vi "Format Container Into String Docs.vi"() -> ()   [LabVIEW 2015]
panel:
  out "resulting string":string
  out "resulting string":string
  out "error out":errorcluster
  out "resulting string":string
  out "resulting string":string
  out "resulting string":string
  out "resulting string":string
  out "resulting string":string
  out "resulting string":string
  out "resulting string":string
  out "resulting string":string
  out "resulting string":string
  out "resulting string":string
  out "resulting string":string
  out "resulting string":string
  out "resulting string":string
  out "resulting string":string
  out "resulting string":string
  out "resulting string":string
  out "resulting string":string
  out "resulting string":string
  out "resulting string":string
  out "resulting string":string
  out "resulting string":string
  out "resulting string":string
  out "resulting string":string
  out "resulting string":string
  out "resulting string":string
  out "resulting string":string
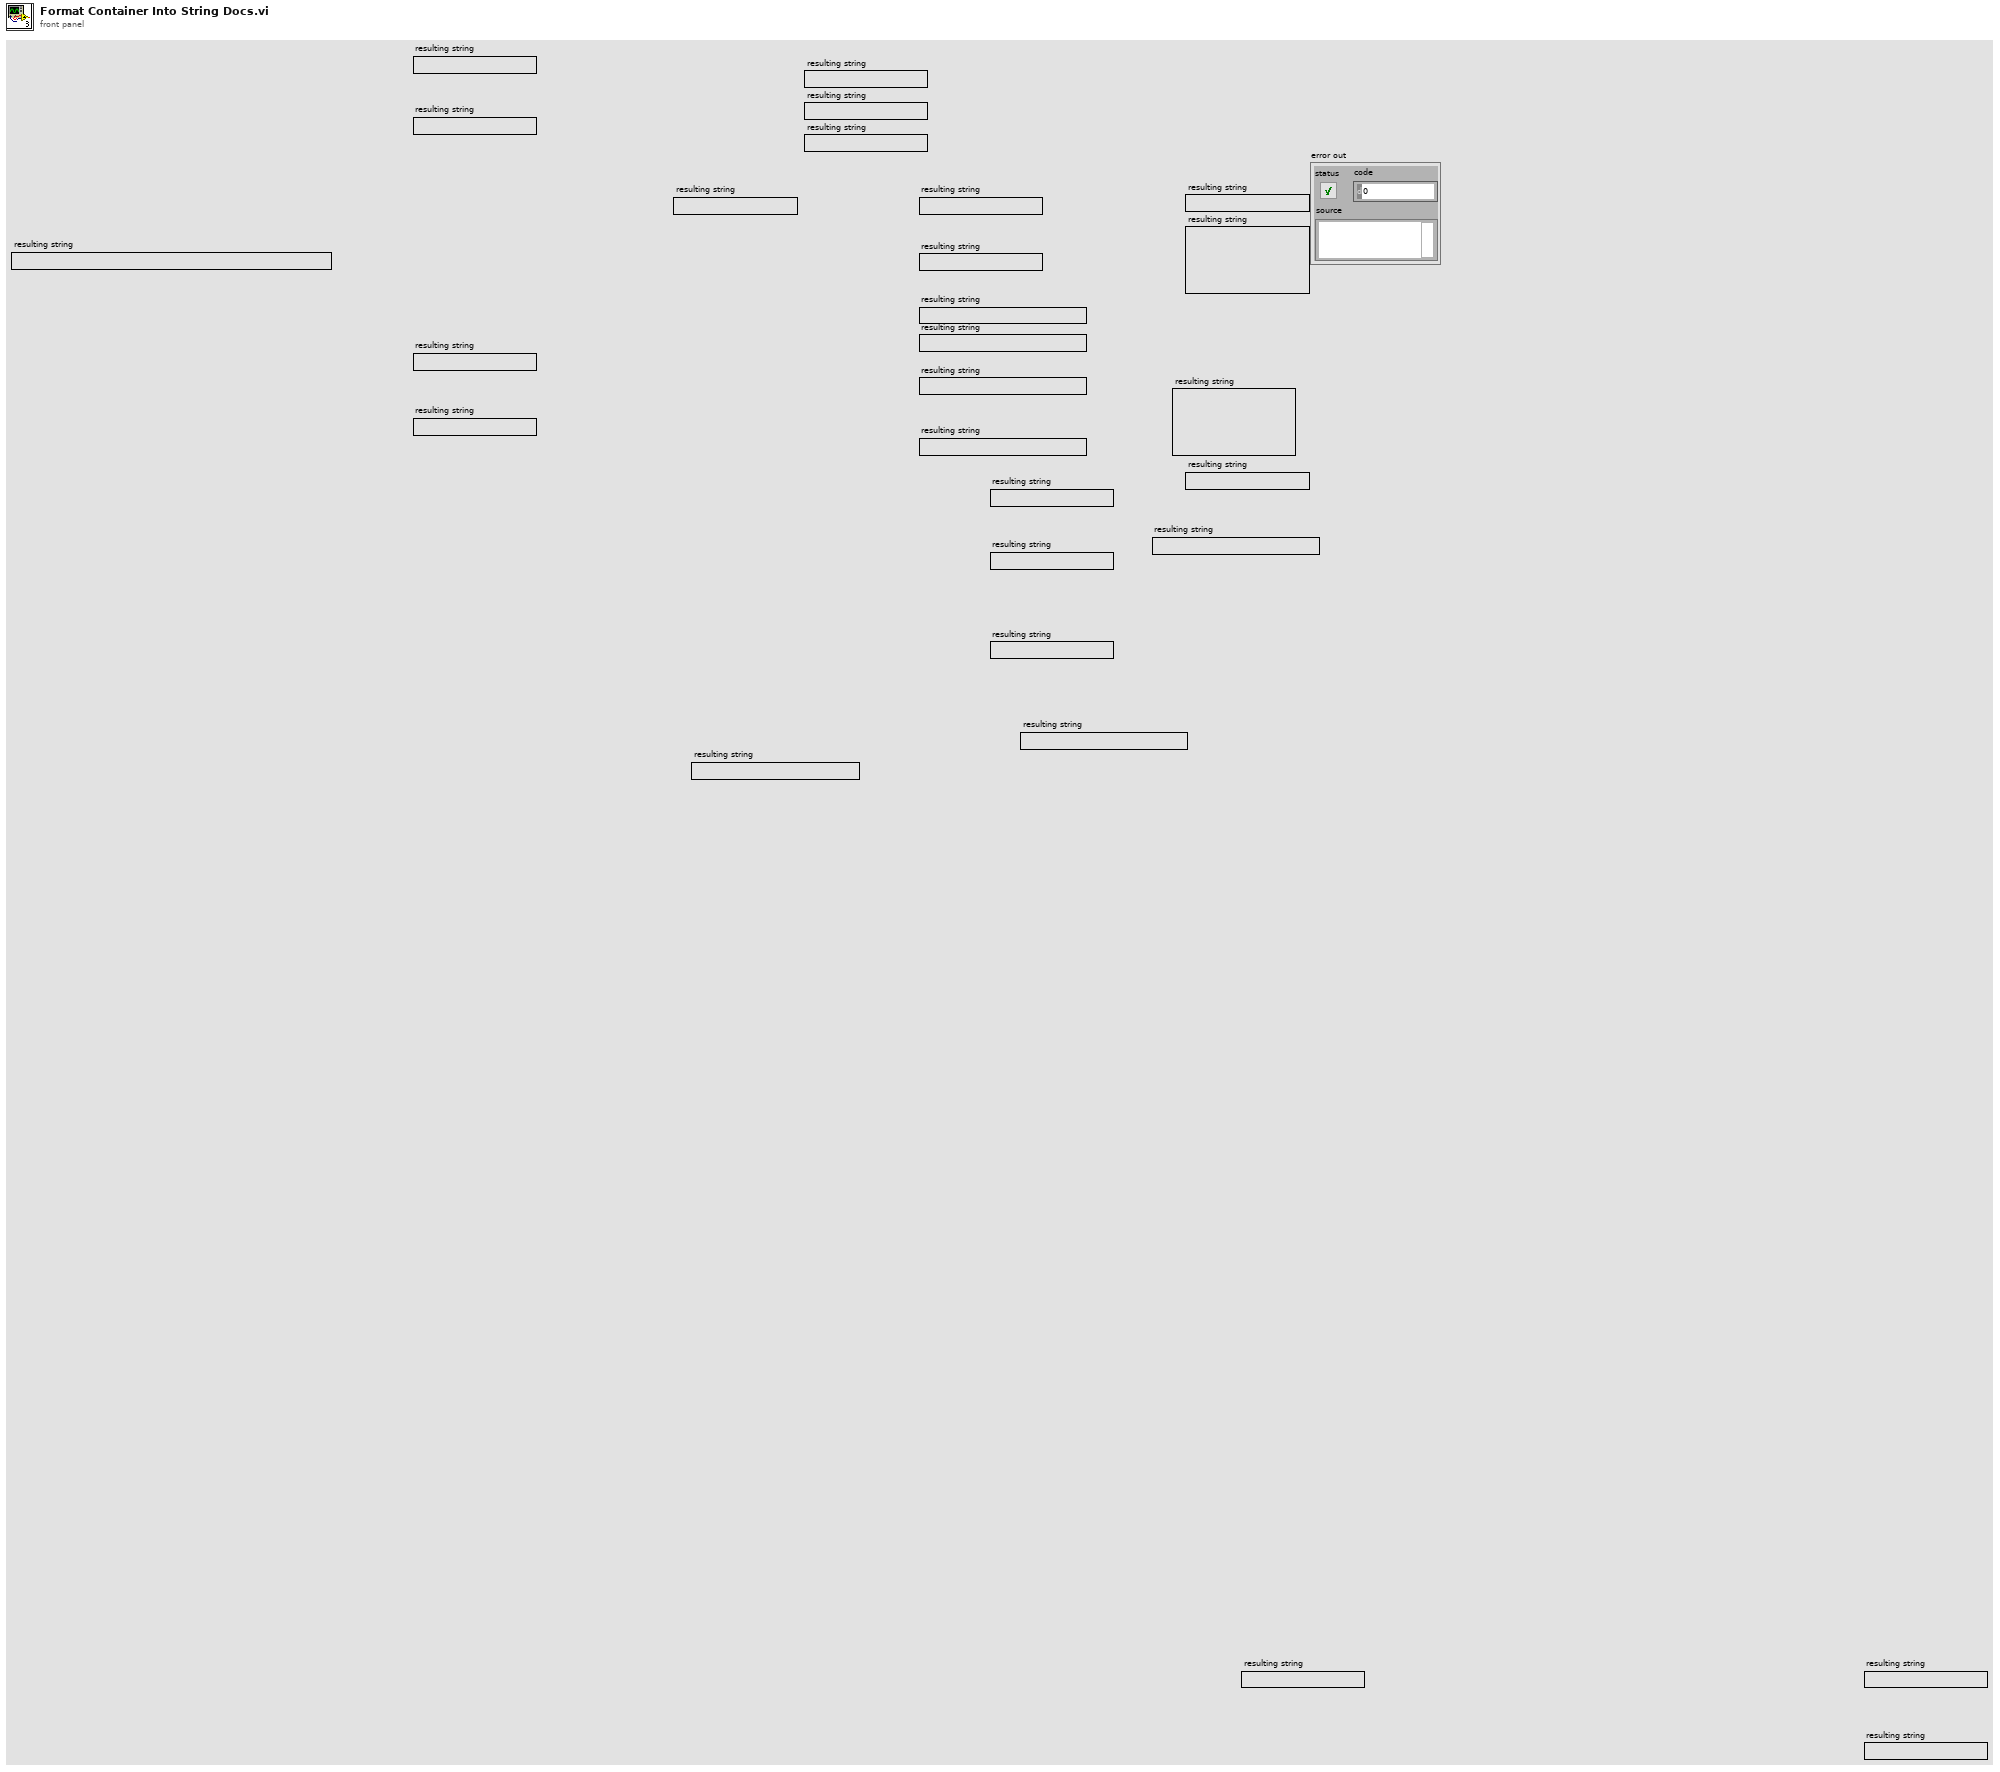
[diagram p1: front panel]
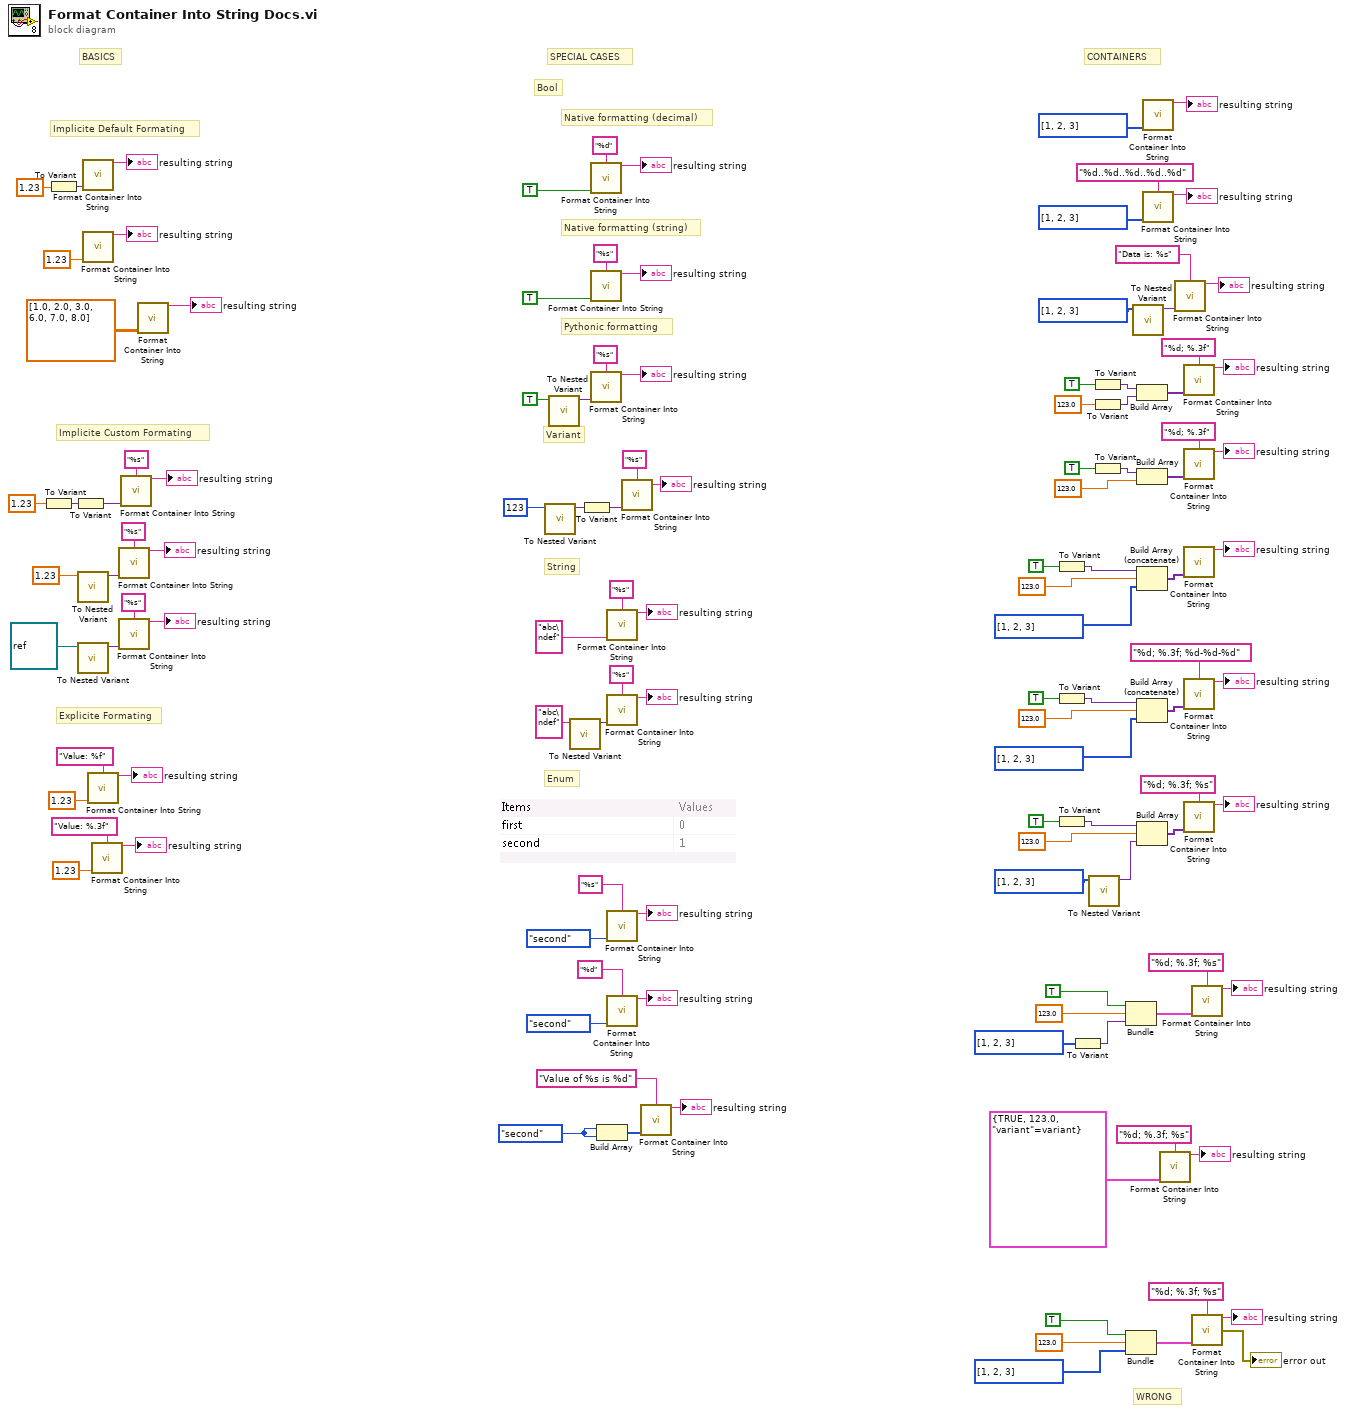
[diagram p0: block diagram]
diagram:
  w2 = enum32{"first", "second"}."second"
  # "Explicite Formating"
  # "Implicite Custom Formating"
  # "Implicite Default Formating"
  # "WRONG"
  # "Bool"
  # "String"
  # "Enum"
  # "Variant"
  # "Pythonic formatting"
  # "Native formatting (decimal)"
  # "Native formatting (string)"
  # "SPECIAL CASES"
  # "CONTAINERS"
  # "BASICS"
  n1 = To Variant(anything=1.23) -> (Variant=w116:variant)
  n2 = To Variant(anything=1.23) -> (Variant=w97:variant)
  n3 = To Variant(anything=w116) -> (Variant=w110:variant)
  n4 = call "To Nested Variant.vi"("variant in"=1.23) -> ("variant out"=w108:variant)  [unwired: 10 in]
  n5 = call "To Nested Variant.vi"("variant in"=refnum<class> refnum ("object")) -> ("variant out"=w73:variant)  [unwired: 10 in]
  n6 = call "Format Container Into String.vi"("input"=w97) -> ("resulting string"=→"resulting string":string)  [unwired: 13 in, 1 out]
  n7 = call "Format Container Into String.vi"("input"=1.23) -> ("resulting string"=→"resulting string":string)  [unwired: 13 in, 1 out]
  n8 = call "Format Container Into String.vi"("format string"="Value: %f", "input"=1.23) -> ("resulting string"=→"resulting string":string)  [unwired: 12 in, 1 out]
  n9 = call "Format Container Into String.vi"("format string"="Value: %.3f", "input"=1.23) -> ("resulting string"=→"resulting string":string)  [unwired: 12 in, 1 out]
  n10 = call "Format Container Into String.vi"("format string"="%s", "input"=w108) -> ("resulting string"=→"resulting string":string)  [unwired: 12 in, 1 out]
  n11 = call "Format Container Into String.vi"("format string"="%s", "input"=w73) -> ("resulting string"=→"resulting string":string)  [unwired: 12 in, 1 out]
  n12 = call "Format Container Into String.vi"("format string"="%s", "input"=w110) -> ("resulting string"=→"resulting string":string)  [unwired: 12 in, 1 out]
  n13 = call "Format Container Into String.vi"("input"=dbl[][] [[1.0, 2.0, 3.0], [6.0, 7.0, 8.0]]) -> ("resulting string"=→"resulting string":string)  [unwired: 13 in, 1 out]
  n14 = call "To Nested Variant.vi"("variant in"=123) -> ("variant out"=w86:variant)  [unwired: 10 in]
  n15 = call "To Nested Variant.vi"("variant in"=TRUE) -> ("variant out"=w90:variant)  [unwired: 10 in]
  n16 = call "To Nested Variant.vi"("variant in"="abc\ndef" ("format string")) -> ("variant out"=w36:variant)  [unwired: 10 in]
  n17 = To Variant(anything=w86) -> (Variant=w84:variant)
  n18 = call "Format Container Into String.vi"("format string"="%d", "input"=TRUE) -> ("resulting string"=→"resulting string":string)  [unwired: 12 in, 1 out]
  n19 = call "Format Container Into String.vi"("format string"="%s", "input"=TRUE) -> ("resulting string"=→"resulting string":string)  [unwired: 12 in, 1 out]
  n20 = call "Format Container Into String.vi"("format string"="%s", "input"=w90) -> ("resulting string"=→"resulting string":string)  [unwired: 12 in, 1 out]
  n21 = Build Array(w2, w2) -> (w3:enum32{"first", "second"}[])
  n22 = call "Format Container Into String.vi"("format string"="%s", "input"="abc\ndef" ("format string")) -> ("resulting string"=→"resulting string":string)  [unwired: 12 in, 1 out]
  n23 = call "Format Container Into String.vi"("format string"="%s", "input"=w36) -> ("resulting string"=→"resulting string":string)  [unwired: 12 in, 1 out]
  n24 = call "Format Container Into String.vi"("format string"="%s", "input"=enum32{"first", "second"}."second") -> ("resulting string"=→"resulting string":string)  [unwired: 12 in, 1 out]
  n25 = call "Format Container Into String.vi"("format string"="%d", "input"=enum32{"first", "second"}."second") -> ("resulting string"=→"resulting string":string)  [unwired: 12 in, 1 out]
  n26 = call "Format Container Into String.vi"("format string"="%s", "input"=w84) -> ("resulting string"=→"resulting string":string)  [unwired: 12 in, 1 out]
  n27 = call "Format Container Into String.vi"("format string"="Value of %s is %d", "input"=w3) -> ("resulting string"=→"resulting string":string)  [unwired: 12 in, 1 out]
  n28 = To Variant(anything=TRUE) -> (Variant=w18:variant)
  n29 = To Variant(anything=TRUE) -> (Variant=w7:variant)
  n30 = To Variant(anything=TRUE) -> (Variant=w45:variant)
  n31 = To Variant(anything=i32[] [1, 2, 3]) -> (Variant=w29:variant)
  n32 = call "To Nested Variant.vi"("variant in"=i32[] [1, 2, 3]) -> ("variant out"=w43:variant)  [unwired: 10 in]
  n33 = To Variant(anything=TRUE) -> (Variant=w57:variant)
  n34 = To Variant(anything=123.0) -> (Variant=w58:variant)
  n35 = To Variant(anything=TRUE) -> (Variant=w56:variant)
  n36 = Bundle(TRUE, 123.0, "Variant"=w29) -> (w33:cluster{bool, dbl, "Variant":variant})  [unwired: 1 in]
  n37 = Bundle(TRUE, 123.0, i32[] [1, 2, 3]) -> (w23:cluster{bool, dbl, i32[]})  [unwired: 1 in]
  n38 = call "To Nested Variant.vi"("variant in"=i32[] [1, 2, 3]) -> ("variant out"=w64:variant)  [unwired: 10 in]
  n39 = Build Array(w57, w58) -> (w63:variant[])
  n40 = Build Array(w56, 123.0) -> (w52:variant[])
  n41 = Build Array (concatenate)(w18, 123.0, i32[] [1, 2, 3]) -> (w15:variant[])
  n42 = Build Array (concatenate)(w7, 123.0, i32[] [1, 2, 3]) -> (w10:variant[])
  n43 = Build Array(w45, 123.0, w43) -> (w49:variant[])
  n44 = call "Format Container Into String.vi"("input"=i32[] [1, 2, 3]) -> ("resulting string"=→"resulting string":string)  [unwired: 13 in, 1 out]
  n45 = call "Format Container Into String.vi"("format string"="%d..%d..%d..%d..%d", "input"=i32[] [1, 2, 3]) -> ("resulting string"=→"resulting string":string)  [unwired: 12 in, 1 out]
  n46 = call "Format Container Into String.vi"("format string"="%d; %.3f; %s", "input"=cluster{bool, dbl, "variant":variant} {TRUE, 123.0, "variant"=variant(i32[] [1, 2, 3])}) -> ("resulting string"=→"resulting string":string)  [unwired: 12 in, 1 out]
  n47 = call "Format Container Into String.vi"("format string"="Data is: %s", "input"=w64) -> ("resulting string"=→"resulting string":string)  [unwired: 12 in, 1 out]
  n48 = call "Format Container Into String.vi"("format string"="%d; %.3f", "input"=w63) -> ("resulting string"=→"resulting string":string)  [unwired: 12 in, 1 out]
  n49 = call "Format Container Into String.vi"("format string"="%d; %.3f", "input"=w52) -> ("resulting string"=→"resulting string":string)  [unwired: 12 in, 1 out]
  n50 = call "Format Container Into String.vi"("input"=w15) -> ("resulting string"=→"resulting string":string)  [unwired: 13 in, 1 out]
  n51 = call "Format Container Into String.vi"("format string"="%d; %.3f; %d-%d-%d", "input"=w10) -> ("resulting string"=→"resulting string":string)  [unwired: 12 in, 1 out]
  n52 = call "Format Container Into String.vi"("format string"="%d; %.3f; %s", "input"=w49) -> ("resulting string"=→"resulting string":string)  [unwired: 12 in, 1 out]
  n53 = call "Format Container Into String.vi"("format string"="%d; %.3f; %s", "input"=w33) -> ("resulting string"=→"resulting string":string)  [unwired: 12 in, 1 out]
  n54 = call "Format Container Into String.vi"("format string"="%d; %.3f; %s", "input"=w23) -> ("resulting string"=→"resulting string":string, "error out"=→"error out":errorcluster)  [unwired: 12 in]
